vi "Get Waveforms.vi"() -> (0 "FFT":picture, 1 "Waveforms":picture)   [LabVIEW 2025, in "MCP Demo Application.lvlib"]
doc: "Returns 3 channels of measurement data and the corresponding FFTs. Use the FFT to characterize the noise level in a channel."
uses:
  MCP Demo Application.lvlib
  Globals.vi
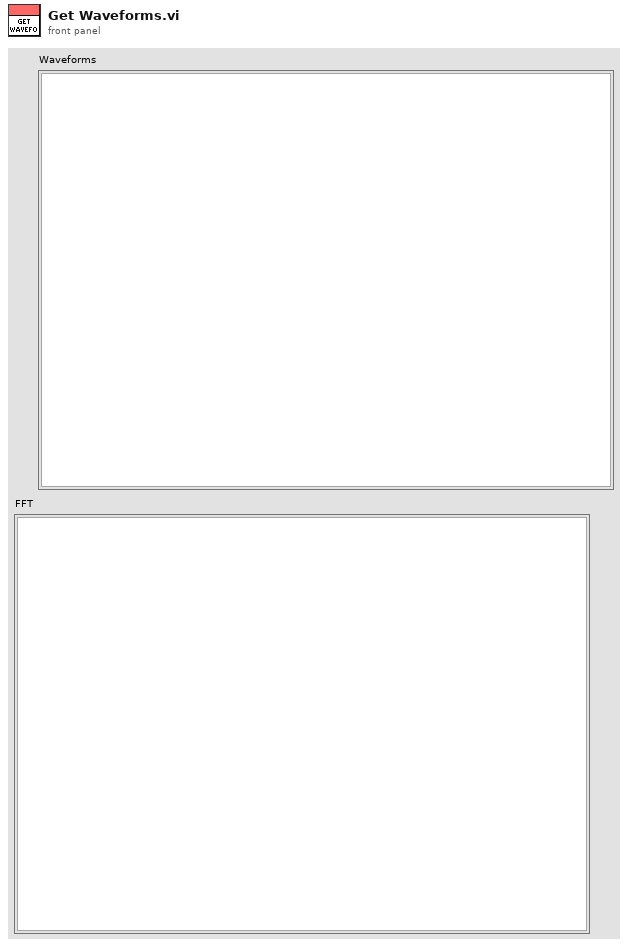
[diagram p1: front panel]
types:
  T1 = typedef "imagedata.ctl" = cluster{"image type":i32, "image depth":i32, "image":u8[], "mask":u8[], "colors":u32[], "Rectangle":cluster{"left":i16, "top":i16, "right":i16, "bottom":i16}}
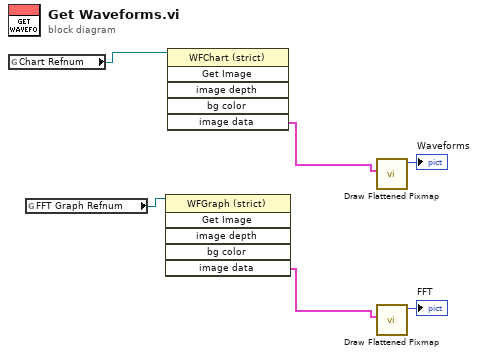
[diagram p0: block diagram]
diagram:
  n1 = global read "Globals.vi" "Chart Refnum"() -> (w5:refnum<vi>)
  n2 = global read "Globals.vi" "FFT Graph Refnum"() -> (w1:refnum<vi>)
  n3 = invoke class="WFGraph (strict)" method="Get Image"(reference=w1) -> ("image data"=w3:T1)  [unwired: 5 in, 5 out]
  n4 = invoke class="WFChart (strict)" method="Get Image"(reference=w5) -> ("image data"=w4:T1)  [unwired: 5 in, 5 out]
  n5 = call <vilib>:"Draw Flattened Pixmap.vi"("image data"=w4) -> ("new picture"=→"Waveforms":picture)  [unwired: 8 in]
  n6 = call <vilib>:"Draw Flattened Pixmap.vi"("image data"=w3) -> ("new picture"=→"FFT":picture)  [unwired: 8 in]
